vi "Receive Message.vi"(6 "priority":i32, 10 "Monitored Actor in":refnum<class "Monitored Actor.lvclass">, 11 "Message in":refnum<class "Message.lvclass">) -> (0 "error out":errorcluster, 2 "Actor out":refnum<class "Actor.lvclass">)   [LabVIEW 2020, in "Monitored Actor.lvlib" / "Monitored Actor.lvclass"]
doc: "This VI should be overriden ONLY if you are creating a proxy actor for remote transmission. If you are, override this VI to transmit the received message to a new destination, maintaining the given priority."
uses:
  <vilib>/MGI/Monitored Actor/Monitored Actor/Monitored Actor/Monitored Actor.lvclass
  <vilib>/ActorFramework/Message/Message.lvclass
  <vilib>/ActorFramework/Actor/Actor.lvclass
  C:/Program Files/National Instruments/LabVIEW 2020/vi.lib/ActorFramework/Actor/Actor.lvclass
  <vilib>/MGI/Monitored Actor/Monitored Actor/Monitored Actor/Monitored Actor.lvclass/Monitored Actor.ctl
  <vilib>/ActorFramework/Actor/Actor.lvclass/Actor.ctl
  <vilib>/ActorFramework/Message Enqueuer/Message Enqueuer.lvclass/Message Enqueuer.ctl
  <vilib>/ActorFramework/Message Enqueuer/Init from Existing Queue.vi
  <vilib>/ActorFramework/Message Enqueuer/Message Enqueuer.lvclass
  <vilib>/MGI/Monitored Actor/Actor Monitor/Actor Monitor Messages/Log Message Msg/Log Message Msg.lvclass
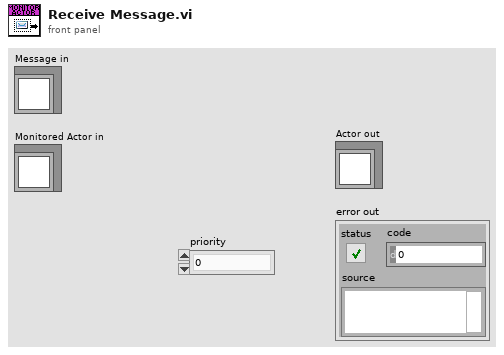
[diagram p1: front panel]
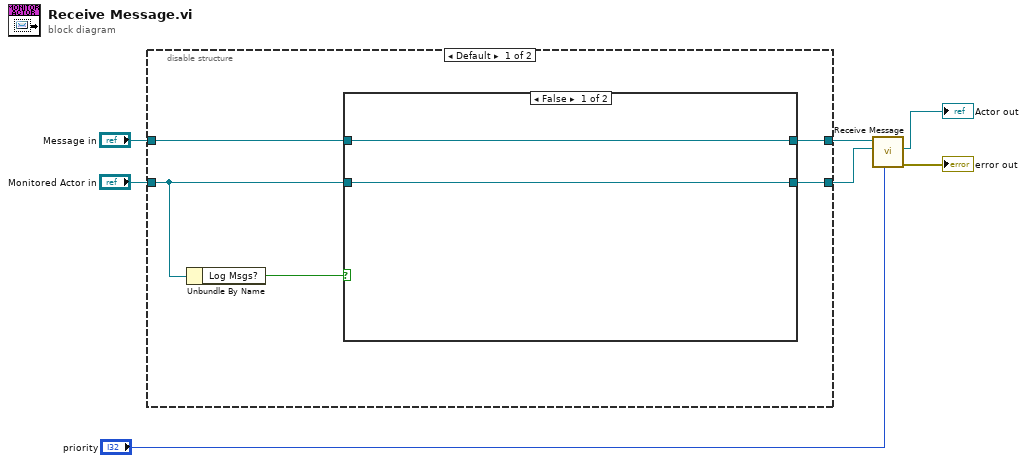
[diagram p0: block diagram]
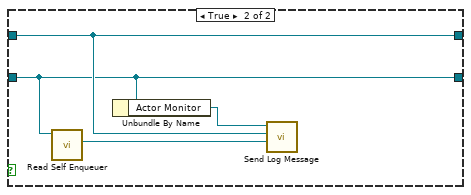
[diagram p2: hidden frame]
diagram:
  n1 = disable-structure shown="Default" {
    disable-tunnel: "Message in" -> [w11 w20]
    disable-tunnel: "Monitored Actor in" -> [w10 w19]
    disable-tunnel: [w9 w20] -> w3
    disable-tunnel: [w8 w19] -> w2
    frame condition #0 (active) {
      n2 = Unbundle By Name(w10) -> ("Log Msgs?"=w12:bool)
      n3 = case shown="False" w12 {
        tunnel: w10 -> [w13 w16]
        tunnel: w11 -> [w14 w17]
        tunnel: [w14 w17] -> w9
        tunnel: [w13 w16] -> w8
        frame False {
        }
        frame True {
          n4 = call <vilib>:"Read Self Enqueuer.vi"("Actor"=w16) -> ("Self Enqueuer"=w18:refnum<class "Message Enqueuer.lvclass">)  [unwired: 10 in]
          n5 = Unbundle By Name(w16) -> ("Actor Monitor"=w15:refnum<class "Message Enqueuer.lvclass">)
          n6 = call <vilib>:"Send Log Message.vi"("Receiving Actor"=w18, "Message"=w17, "Message Enqueuer in"=w15) -> ()  [unwired: 7 in, 2 out]
        }
      }
    }
    frame condition #1 {
    }
  }
  n7 = call-parent "Receive Message.vi"("priority"="priority", "Actor in"=w2, "Message in"=w3) -> ("error out"=→"error out":errorcluster, "Actor out"=→"Actor out":refnum<class "Actor.lvclass">)  [unwired: 7 in]
